vi "DSP_WriteRAM.vi"(2 "error in (no error)":errorcluster, 3 "values":u16[](array[numeric]), 4 "Board Handle":u64) -> (0 "error out":errorcluster, 1 "Board Handle Out":u64)   [LabVIEW 2009]
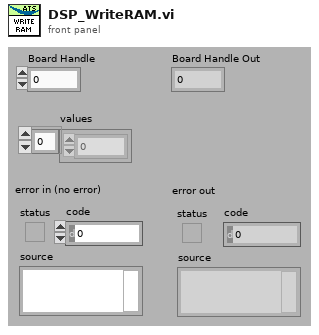
[diagram p1: front panel]
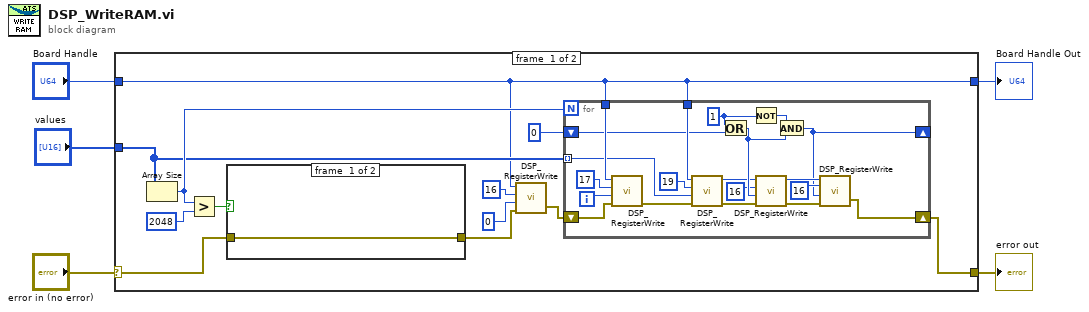
[diagram p0: block diagram]
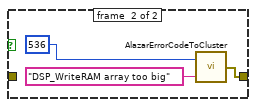
[diagram p2: hidden frame]
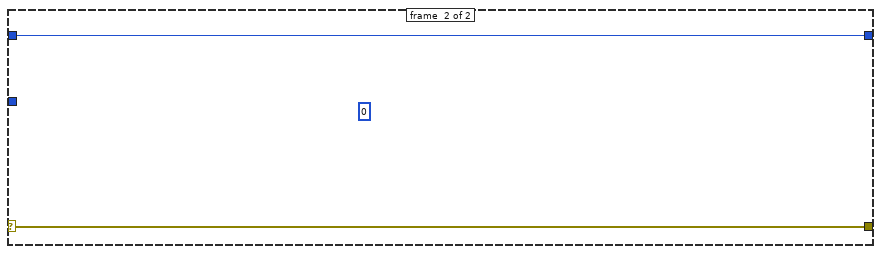
[diagram p3: hidden frame]
diagram:
  n1 = case shown="No Error" "error in (no error)" {
    selector: "error in (no error)" -> [w15 w43]
    tunnel: [w7 w43] -> w4
    tunnel: [w9 w42] -> w3
    tunnel: "Board Handle" -> [w9 w42]
    tunnel: "values" -> [w10 _]
    frame #0 {
      n2 = Array Size(array=w10) -> (size(s)=w12:i32)
      n3 = Greater?(x=w12, y=2048) -> (0:w16:bool)
      n4 = case shown="True" w16 {
        tunnel: w15 -> [w38 _]
        tunnel: [w38 w39] -> w14
        frame #0 {
        }
        frame #1 {
          n5 = call "AlazarErrorCodeToCluster.vi"("Message"="DSP_WriteRAM array too big", "Error Code"=u32 536) -> ("error out"=w39:errorcluster)
        }
      }
      n6 = call "DSP_RegisterWrite.vi"("error in (no error)"=w14, "Value"=u32 0, "Offset"=u32 16, "Board Handle"=w9) -> ("error out"=w11:errorcluster)  [unwired: 1 out]
      n7 = for {
        N: w12 -> [_]
        tunnel: w9 -> [w35]
        shift-right: [w20] -> w7
        shift-left: w11 -> [w34]
        tunnel: w10 -> [w32] mode=indexing
        tunnel: w9 -> [w31]
        shift-right: [w18] -> _
        shift-left: u32 0 -> [w19]
        i -> [w37]
        w28 = u32 1
        n8 = call "DSP_RegisterWrite.vi"("error in (no error)"=w34, "Value"=w37, "Offset"=u32 17, "Board Handle"=w35) -> ("error out"=w30:errorcluster)  [unwired: 1 out]
        n9 = call "DSP_RegisterWrite.vi"("error in (no error)"=w30, "Value"=w32, "Offset"=u32 19, "Board Handle"=w31) -> ("error out"=w24:errorcluster, "Board Handle Out"=w26:u64)
        n10 = Or(x=w28, y=w19) -> (x .or. y?=w27:u32)
        n11 = Not(x=w28) -> (.not. x?=w29:u32)
        n12 = call "DSP_RegisterWrite.vi"("error in (no error)"=w24, "Value"=w27, "Offset"=u32 16, "Board Handle"=w26) -> ("error out"=w23:errorcluster, "Board Handle Out"=w25:u64)
        n13 = And(x=w29, y=w27) -> (x .and. y?=w18:u32)
        n14 = call "DSP_RegisterWrite.vi"("error in (no error)"=w23, "Value"=w18, "Offset"=u32 16, "Board Handle"=w25) -> ("error out"=w20:errorcluster)  [unwired: 1 out]
      }
    }
    frame #1 {
      (unwired) u32 0
    }
  }
  "Board Handle Out" <- w3
  "error out" <- w4
